vi "Simulator.vi"(4 "T_max":dbl=33.5, 6 "T_min":dbl=20.5, 8 "Q_kulso_0":dbl, 9 "mód":enum16{"szinusz", "ugrás"}(ring), 10 "Parameterek in":T2, 11 "t_sim [nap]":dbl) -> (2 "output cluster":T1)   [LabVIEW 2013]
uses:
  Parameterek.ctl
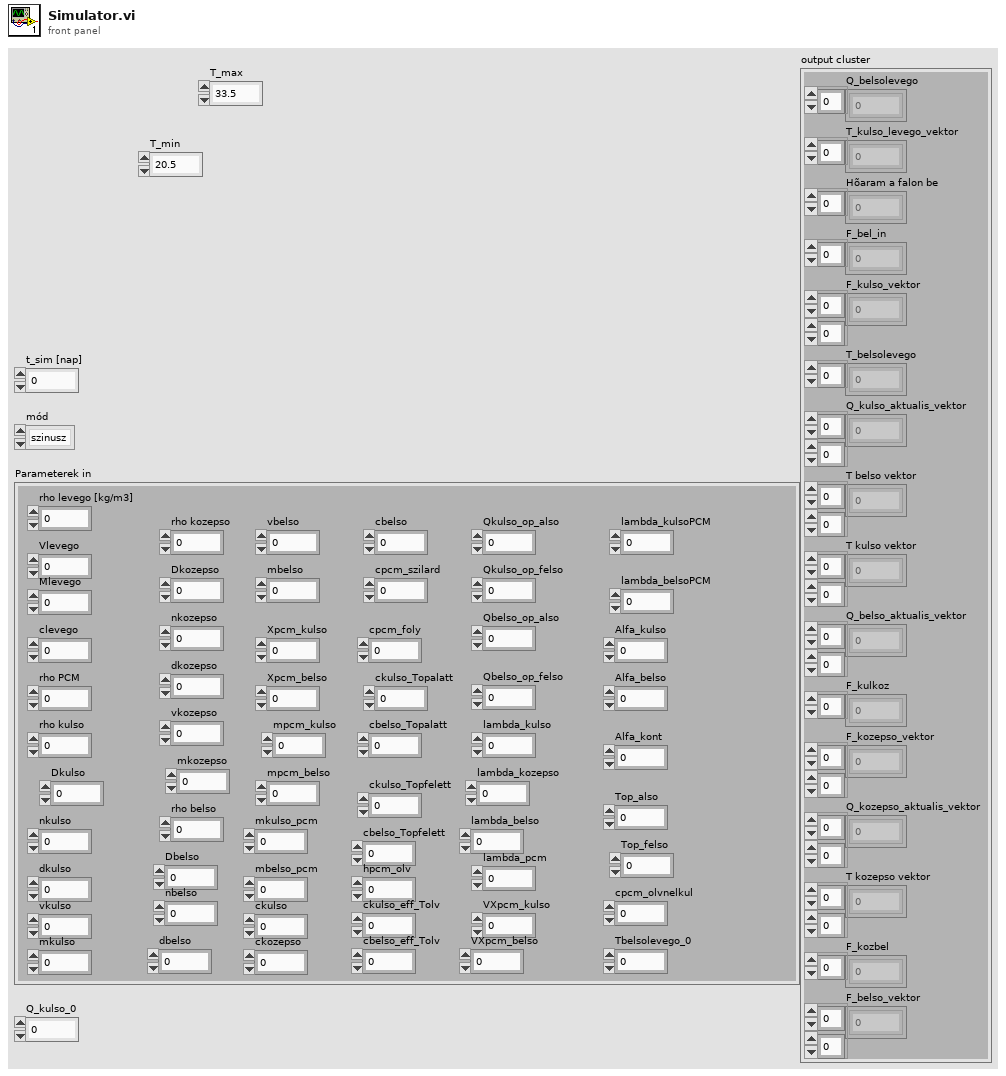
[diagram p1: front panel]
types:
  T1 = cluster{"Q_belsolevego":dbl[], "T_kulso_levego_vektor":dbl[], "Hõaram a falon be":dbl[], "F_bel_in":dbl[], "F_kulso_vektor":dbl[][], "T_belsolevego":dbl[], "Q_kulso_aktualis_vektor":dbl[][], "T belso vektor":dbl[][], "T kulso vektor":dbl[][], "Q_belso_aktualis_vektor":dbl[][], "F_kulkoz":dbl[], "F_kozepso_vektor":dbl[][], "Q_kozepso_aktualis_vektor":dbl[][], "T kozepso vektor":dbl[][], "F_kozbel":dbl[], "F_belso_vektor":dbl[][]}
  T2 = typedef "Parameterek.ctl" = cluster{"rholevego":dbl, "Vlevego":dbl, "Mlevego":dbl, "clevego":dbl, "rho PCM":dbl, "rho kulso":dbl, "Dkulso":dbl, "nkulso":i32, "dkulso":dbl, "vkulso":dbl, "rho kozepso":dbl, "Dkozepso":dbl, "nkozepso":i32, "dkozepso":dbl, "vkozepso":dbl, "mkozepso":dbl, "mkulso":dbl, "rho belso":dbl, "Dbelso":dbl, "nbelso":i32, "dbelso":dbl, "vbelso":dbl, "mbelso":dbl, "Xpcm_kulso":dbl, "Xpcm_belso":dbl, "mpcm_kulso":dbl, "mpcm_belso":dbl, "mkulso_pcm":dbl, "mbelso_pcm":dbl, "ckulso":dbl, "ckozepso":dbl, "cbelso":dbl, "cpcm_szilard":dbl, "cpcm_foly":dbl, "ckulso_Topalatt":dbl, "cbelso_Topalatt":dbl, "ckulso_Topfelett":dbl, "cbelso_Topfelett":dbl, "hpcm_olv":dbl, "ckulso_eff_Tolv":dbl, "cbelso_eff_Tolv":dbl, "Qkulso_op_also":dbl, "Qkulso_op_felso":dbl, "Qbelso_op_also":dbl, "Qbelso_op_felso":dbl, "lambda_kulso":dbl, "lambda_kozepso":dbl, "lambda_belso":dbl, "lambda_pcm":dbl, "VXpcm_kulso":dbl, "VXpcm_belso":dbl, "lambda_kulsoPCM":dbl, "lambda_belsoPCM":dbl, "Alfa_kulso":dbl, "Alfa_belso":dbl, "Alfa_kont":dbl, "Top_also":dbl, "Top_felso":dbl, "cpcm_olvnelkul":dbl, "Tbelsolevego_0":dbl}
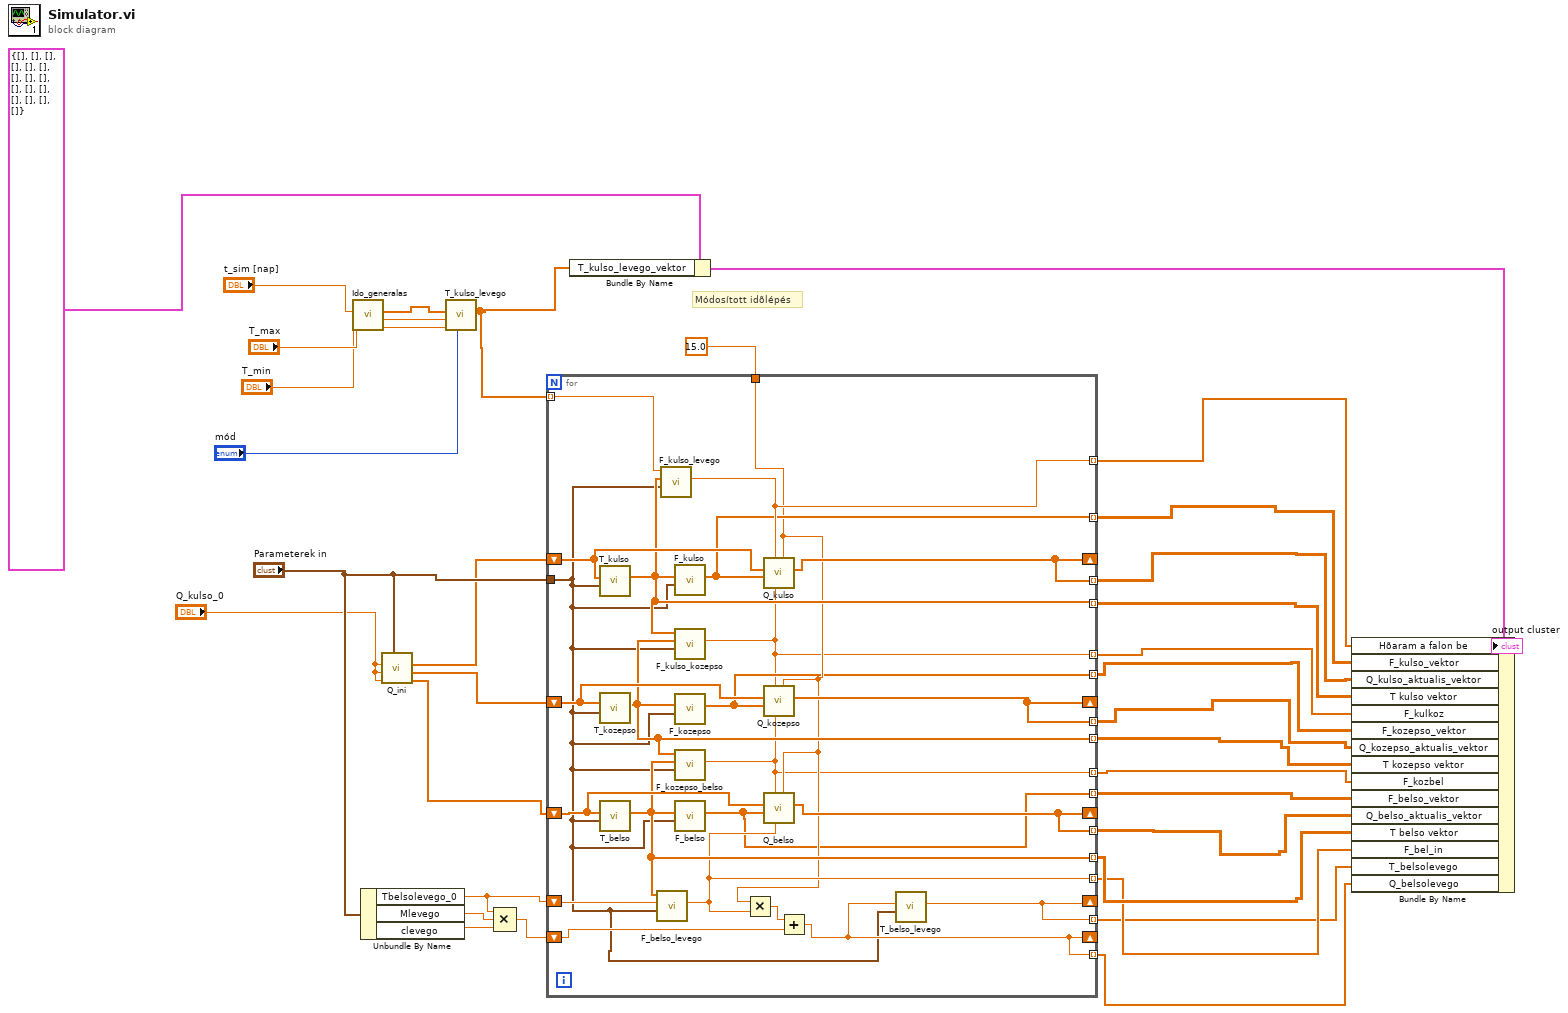
[diagram p0: block diagram]
diagram:
  # "Módosított idõlépés"
  n1 = call "Ido_generalas.vi"("t_sim [nap]"="t_sim [nap]") -> ("t_vektor"=w32:dbl[])  [unwired: 10 in]
  n2 = Unbundle By Name("Parameterek in") -> ("Tbelsolevego_0"=w28:dbl, "Mlevego"=w30:dbl, "clevego"=w31:dbl)
  n3 = call "Q_ini.vi"("Parameterek"="Parameterek in", "T_belso_0"="Q_kulso_0", "T_kozepso_0"="Q_kulso_0", "T_kulso_0"="Q_kulso_0") -> ("Q_belso_0_vektor"=w26:dbl[], "Q_kozepso_0_vektor"=w25:dbl[], "Q_kulso_0 vektor"=w24:dbl[])  [unwired: 5 in]
  n4 = call "T_kulso_levego.vi"("mód"="mód", "T_min"="T_min", "T_max"="T_max", "t_vektor"=w32) -> ("T_kulso_levego_vektor"=w21:dbl[])  [unwired: 6 in, 1 out]
  n5 = Compound Arithmetic op=MULTIPLY(w28, w30, w31) -> (w27:dbl)
  n6 = for {
    tunnel: w21 -> [w57] mode=indexing
    shift-right: [w56] -> _
    shift-left: w25 -> [w58]
    tunnel: [w56] -> w12 mode=indexing
    tunnel: [w50] -> w11 mode=indexing
    tunnel: "Parameterek in" -> [w40]
    shift-right: [w54] -> _
    shift-left: w24 -> [w55]
    shift-right: [w52] -> _
    shift-left: w26 -> [w53]
    tunnel: [w54] -> w16 mode=indexing
    tunnel: [w51] -> w15 mode=indexing
    tunnel: [w52] -> w8 mode=indexing
    tunnel: [w49] -> w7 mode=indexing
    shift-right: [w45] -> _
    shift-left: w28 -> [w48]
    shift-right: [w44] -> _
    shift-left: w27 -> [w47]
    tunnel: [w45] -> w5 mode=indexing
    tunnel: [w44] -> w4 mode=indexing
    tunnel: [w43] -> w18 mode=indexing
    tunnel: [w42] -> w17 mode=indexing
    tunnel: [w36] -> w14 mode=indexing
    tunnel: [w35] -> w10 mode=indexing
    tunnel: [w41] -> w6 mode=indexing
    tunnel: 15.0 ("dt") -> [w39]
    tunnel: [w38] -> w13 mode=indexing
    tunnel: [w37] -> w9 mode=indexing
    n7 = call "T_kulso.vi"("Parameterek"=w40, "Q kulso vektor"=w55) -> ("T kulso vektor"=w51:dbl[])  [unwired: 9 in]
    n8 = call "T_kozepso.vi"("Parameterek"=w40, "Q kozepso vektor"=w58) -> ("T kozepso vektor"=w50:dbl[])  [unwired: 9 in]
    n9 = call "T_belso.vi"("Parameterek"=w40, "Q belso vektor"=w53) -> ("T belso vektor"=w49:dbl[])  [unwired: 9 in]
    n10 = call "F_belso_levego.vi"("Parameterek"=w40, "T_belso_levego"=w48, "T_belso_vektor"=w49) -> ("F_fal_belso_levego"=w41:dbl)  [unwired: 8 in]
    n11 = call "F_kulso_levego.vi"("Parameterek"=w40, "T_kulso_vektor"=w51, "T_kulso_levego"=w57) -> ("F_kulso_levego_fal"=w43:dbl)  [unwired: 8 in]
    n12 = call "F_kulso.vi"("Parameterek"=w40, "T_kulso_vektor"=w51) -> ("F_kulso_vektor"=w42:dbl[])  [unwired: 9 in]
    n13 = call "F_kulso_kozepso.vi"("T_kulso_vektor"=w51, "T_kozepso_vektor"=w50, "Parameterek"=w40) -> ("F_10_11"=w36:dbl)  [unwired: 7 in]
    n14 = call "F_kozepso.vi"("Parameterek"=w40, "T_kozepso_vektor"=w50) -> ("F_kozepso_vektor"=w38:dbl[])  [unwired: 9 in]
    n15 = call "F_kozepso_belso.vi"("T_kozepso_vektor"=w50, "T_belso_vektor"=w49, "Parameterek"=w40) -> ("F_16_17"=w35:dbl)  [unwired: 7 in]
    n16 = call "F_belso.vi"("Parameterek"=w40, "T_belso_vektor"=w49) -> ("F_belso_vektor"=w37:dbl[])  [unwired: 9 in]
    n17 = Multiply(x=w39, y=w41) -> (x*y=w46:dbl)
    n18 = call "Q_kulso.vi"("idolepes"=w39, "F_10_11"=w36, "F_kulso_levego_fal"=w43, "F_kulso_vektor"=w42, "Q_kulso_elozo_vektor"=w55) -> ("Q_kulso_aktualis_vektor"=w54:dbl[])  [unwired: 6 in]
    n19 = call "Q_kozepso.vi"("idolepes"=w39, "F_kozbel"=w35, "F_kulkoz"=w36, "F_kozepso_vektor"=w38, "Q_kozepso_elozo_vektor"=w58) -> ("Q_kozepso_aktualis_vektor"=w56:dbl[])  [unwired: 6 in]
    n20 = call "Q_belso.vi"("idolepes"=w39, "F_belso_fal"=w41, "F_16_17"=w35, "F_belso_vektor"=w37, "Q_belso_elozo_vektor"=w53) -> ("Q_belso_aktualis_vektor"=w52:dbl[])  [unwired: 6 in]
    n21 = Add(x=w46, y=w47) -> (x+y=w44:dbl)
    n22 = call "T_belso_levego.vi"("Parameterek"=w40, "Q_belsolevego"=w44) -> ("T_belsolevego"=w45:dbl)  [unwired: 9 in]
  }
  n23 = Bundle By Name(cluster=T1 {"Q_belsolevego"=[], "T_kulso_levego_vektor"=[], "Hõaram a falon be"=[], "F_bel_in"=[], "F_kulso_vektor"=[], "T_belsolevego"=[], "Q_kulso_aktualis_vektor"=[], "T belso vektor"=[], "T kulso vektor"=[], "Q_belso_aktualis_vektor"=[], "F_kulkoz"=[], "F_kozepso_vektor"=[], "Q_kozepso_aktualis_vektor"=[], "T kozepso vektor"=[], "F_kozbel"=[], "F_belso_vektor"=[]} ("Output"), "T_kulso_levego_vektor"=w21) -> (w3:T1)
  n24 = Bundle By Name(cluster=w3, "Hõaram a falon be"=w18, "F_kulso_vektor"=w17, "Q_kulso_aktualis_vektor"=w16, "T kulso vektor"=w15, "F_kulkoz"=w14, "F_kozepso_vektor"=w13, "Q_kozepso_aktualis_vektor"=w12, "T kozepso vektor"=w11, "F_kozbel"=w10, "F_belso_vektor"=w9, "Q_belso_aktualis_vektor"=w8, "T belso vektor"=w7, "F_bel_in"=w6, "T_belsolevego"=w5, "Q_belsolevego"=w4) -> (→"output cluster":T1)
